vi "Define End If.vi"(11 "String in":string) -> (3 "String out":string)   [LabVIEW 2014, in "C Header Generator.lvlib"]
uses:
  C Header Generator.lvlib
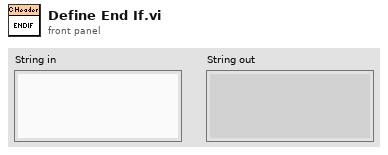
[diagram p1: front panel]
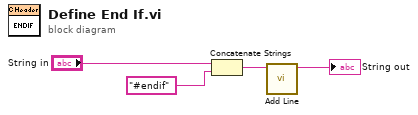
[diagram p0: block diagram]
diagram:
  n1 = Concatenate Strings("String in", "#endif") -> (w2:string)
  n2 = call "Add Line.vi"("String in"=w2) -> ("String out"=→"String out":string)  [unwired: 10 in]
